vi "Method.vi"(4 "Bool":refnum<class "Abs_Boolean.lvclass">) -> (1 "Result":refnum<class "Abs_Boolean.lvclass">)   [LabVIEW 2021, in "NOT_Bool.lvclass"]
uses:
  NOT_Bool.lvclass
  Abs_Types/Boolean/Abs_Boolean.lvclass
  C:/TSA/LV_Abstract/Source/Functions/Support/Function/One Terminal/Boolean/AbsFunc_One Term_Bool.lvclass
  C:/Program Files (x86)/National Instruments/LabVIEW 2021/vi.lib/TSA/Abstract Data Classes/Abs_Types/Boolean/Abs_Boolean.lvclass
  Support/Function/One Terminal/Boolean/AbsFunc_One Term_Bool.lvclass/AbsFunc_One Term_Bool.ctl
  Support/Function/One Terminal/Boolean/Properties/Write Bool A.vi
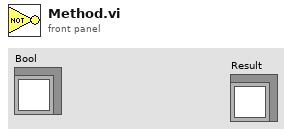
[diagram p1: front panel]
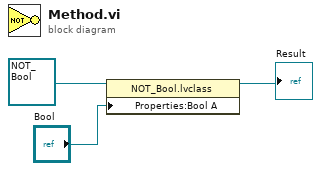
[diagram p0: block diagram]
diagram:
  n1 = property class="NOT_Bool.lvclass"(reference=refnum<class "NOT_Bool.lvclass"> refnum ("Functions.lvlib:Logic.lvlib:NOT.lvclass"), "Properties:Bool A"="Bool") -> (reference out=→"Result":refnum<class "NOT_Bool.lvclass">)  [unwired: 1 in, 1 out]
